vi "gyro encoder safety.vi"(8 "Cutoff Rate":dbl=0.2, 9 "Gyro Angular Rate":dbl, 10 "Encoder Rate":dbl, 11 "Input":dbl) -> (0 "No Gyro Rate Read":bool, 1 "No Encoder Rate Read":bool, 2 "Encoder Failure":bool, 3 "Output":dbl, 4 "Gyro Failure":bool)   [LabVIEW 2014]
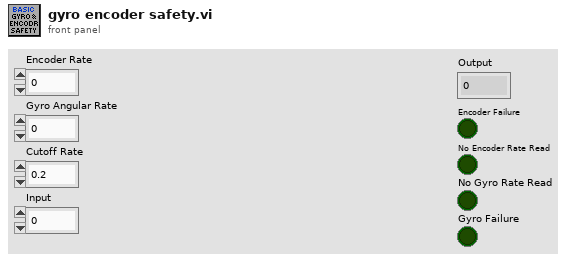
[diagram p1: front panel]
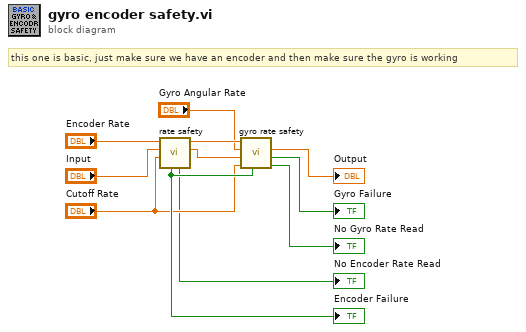
[diagram p0: block diagram]
diagram:
  # "this one is basic, just make sure we have an encoder and then make sure the gyro is working"
  n1 = call "rate safety.vi"("Cutoff Rate"="Cutoff Rate", "Desired Rate"="Input", "Encoder Rate"="Encoder Rate") -> ("Output Rate"=w9:dbl, "Encoder Rate Out"=w11:dbl, "No Rate Read"=→"No Encoder Rate Read":bool, "Encoder Failure"=w10:bool)  [unwired: 5 in]
  "Encoder Failure" <- w10
  n2 = call "gyro rate safety.vi"("Encoder Failure"=w10, "Cutoff Rate"="Cutoff Rate", "Input"=w9, "Gyro Angular Rate"="Gyro Angular Rate", "Encoder Rate"=w11) -> ("No Gyro Rate Read"=→"No Gyro Rate Read":bool, "Gyro Failure"=→"Gyro Failure":bool, "Output"=→"Output":dbl)  [unwired: 3 in, 1 out]
